vi "电源管理UI.vi"() -> ()   [LabVIEW 2016, in "PLC.lvlib"]
uses:
  PLC.lvlib
  <vilib>/Utility/miscctls.llb/LVPointTypeDef.ctl
panel:
  in  "总氮电源":bool
  in  "CODCr电源":bool
  in  "总磷电源":bool
  in  "氨氮电源":bool
  in  "CODMn电源":bool
  in  "多参数电源":bool
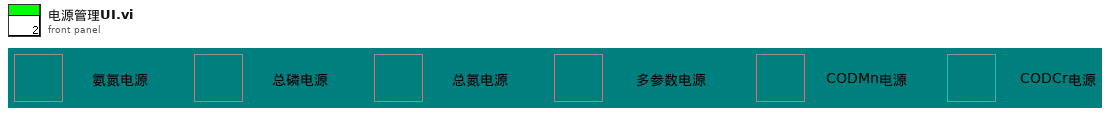
[diagram p1: front panel]
types:
  T1 = typedef "LVPointTypeDef.ctl" = cluster{"Horizontal":i16, "Vertical":i16}
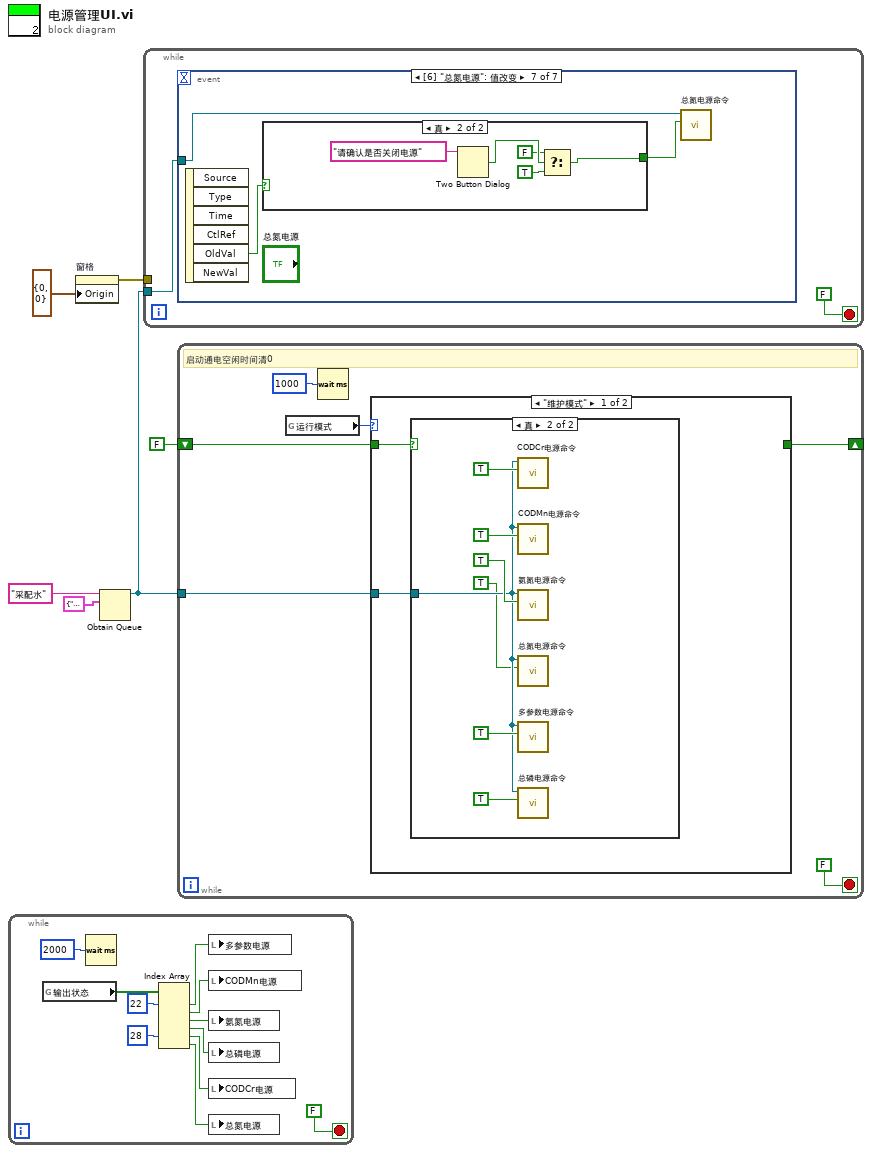
[diagram p0: block diagram]
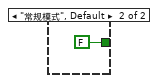
[diagram p3: hidden frame]
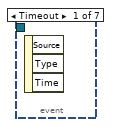
[diagram p4: hidden frame]
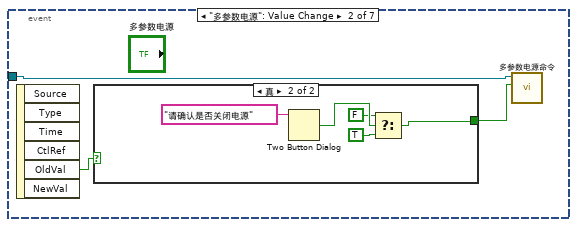
[diagram p5: hidden frame]
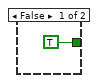
[diagram p6: hidden frame]
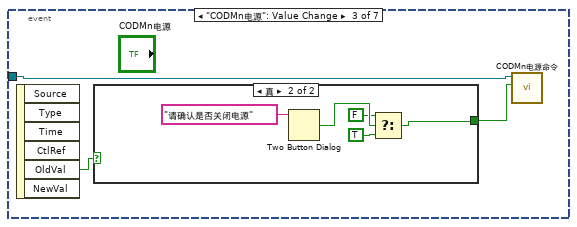
[diagram p7: hidden frame]
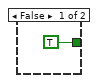
[diagram p8: hidden frame]
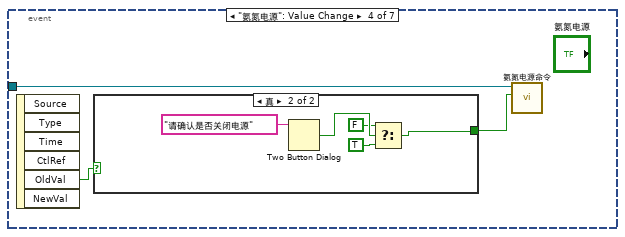
[diagram p9: hidden frame]
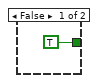
[diagram p10: hidden frame]
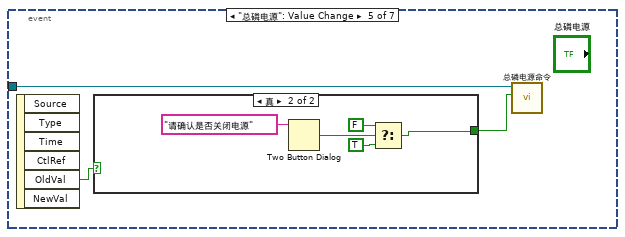
[diagram p11: hidden frame]
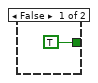
[diagram p12: hidden frame]
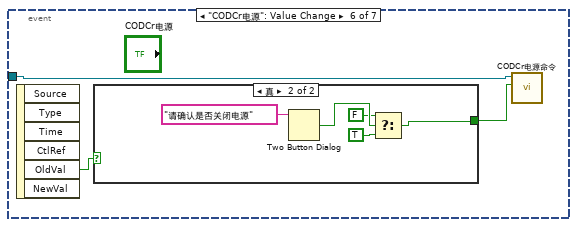
[diagram p13: hidden frame]
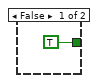
[diagram p14: hidden frame]
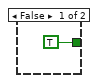
[diagram p15: hidden frame]
diagram:
  n1 = while {
    stop <- FALSE stop-if-true
    n2 = global read "采配水全局变量.vi" "输出状态"() -> (w15:bool[])
    n3 = Wait (ms)(milliseconds to wait=u32 2000 ("等待时间（毫秒）")) -> ()  [unwired: 1 out]
    n4 = Index Array(array=w15, index #1=22 ("索引"), index #5=28 ("索引")) -> (element #1=w10:bool, element #2=w13:bool, element #3=w12:bool, element #4=w11:bool, element #5=w8:bool, element #6=w7:bool)  [unwired: 4 in]
    n5 = local write "多参数电源"(w10) -> ()
    n6 = local write "CODMn电源"(w13) -> ()
    n7 = local write "氨氮电源"(w12) -> ()
    n8 = local write "总磷电源"(w11) -> ()
    n9 = local write "CODCr电源"(w8) -> ()
    n10 = local write "总氮电源"(w7) -> ()
  }
  n11 = property on="窗格" class="Pane"("Origin"=T1 {"Horizontal"=0, "Vertical"=0} ("原点")) -> (error out=w3:errorcluster)  [unwired: 2 in, 1 out]
  n12 = Obtain Queue(name (unnamed)="采配水" ("名称（未命名）"), element data type=cluster{"命令":string, "数据":variant} {"命令"="", "数据"=variant}) -> (queue out=w2:refnum<queue>)  [unwired: 3 in, 2 out]
  n13 = while {
    tunnel: w2 -> [w18]
    tunnel: w3 -> [_]
    stop <- FALSE stop-if-true
    n14 = event shown="[6] \"总氮电源\": 值改变" {
      selector: _ -> [_ _ _ _ _ _ _]
      dyn-events: _ -> [_ _ _ _ _ _ _]
      timeout: _ -> [_ _ _ _ _ _ _]
      tunnel: w18 -> [_ w22 w31 w40 w49 w58 w67]
      event Timeout {
        n15 = event-data() -> ()  [unwired: 1 in, 3 out]
      }
      event "多参数电源": Value Change {
        n16 = event-data() -> ("OldVal"=w21:bool)  [unwired: 1 in, 5 out]
        n17 = case shown="真" w21 {
          tunnel: [TRUE ("T button?") w24] -> w20
          frame False {
          }
          frame True {
            n18 = Two Button Dialog(message="请确认是否关闭电源" ("消息")) -> (T button?=w27:bool)  [unwired: 2 in]
            n19 = Select(t=FALSE, s=w27, f=TRUE ("T button?")) -> (s? t:f=w24:bool)
          }
        }
        n20 = call "多参数电源命令.vi"("通电/断电"=w20, "队列"=w22) -> ()  [unwired: 9 in, 1 out]
      }
      event "CODMn电源": Value Change {
        n21 = event-data() -> ("OldVal"=w30:bool)  [unwired: 1 in, 5 out]
        n22 = case shown="真" w30 {
          tunnel: [TRUE ("T button?") w33] -> w29
          frame False {
          }
          frame True {
            n23 = Two Button Dialog(message="请确认是否关闭电源" ("消息")) -> (T button?=w36:bool)  [unwired: 2 in]
            n24 = Select(t=FALSE, s=w36, f=TRUE ("T button?")) -> (s? t:f=w33:bool)
          }
        }
        n25 = call "CODMn电源命令.vi"("通电/断电"=w29, "队列"=w31) -> ()  [unwired: 9 in, 1 out]
      }
      event "氨氮电源": Value Change {
        n26 = event-data() -> ("OldVal"=w39:bool)  [unwired: 1 in, 5 out]
        n27 = case shown="真" w39 {
          tunnel: [TRUE ("T button?") w42] -> w38
          frame False {
          }
          frame True {
            n28 = Two Button Dialog(message="请确认是否关闭电源" ("消息")) -> (T button?=w45:bool)  [unwired: 2 in]
            n29 = Select(t=FALSE, s=w45, f=TRUE ("T button?")) -> (s? t:f=w42:bool)
          }
        }
        n30 = call "氨氮电源命令.vi"("通电/断电"=w38, "队列"=w40) -> ()  [unwired: 9 in, 1 out]
      }
      event "总磷电源": Value Change {
        n31 = event-data() -> ("OldVal"=w48:bool)  [unwired: 1 in, 5 out]
        n32 = case shown="真" w48 {
          tunnel: [TRUE ("T button?") w51] -> w47
          frame False {
          }
          frame True {
            n33 = Two Button Dialog(message="请确认是否关闭电源" ("消息")) -> (T button?=w54:bool)  [unwired: 2 in]
            n34 = Select(t=FALSE, s=w54, f=TRUE ("T button?")) -> (s? t:f=w51:bool)
          }
        }
        n35 = call "总磷电源命令.vi"("通电/断电"=w47, "队列"=w49) -> ()  [unwired: 9 in, 1 out]
      }
      event "CODCr电源": Value Change {
        n36 = event-data() -> ("OldVal"=w57:bool)  [unwired: 1 in, 5 out]
        n37 = case shown="真" w57 {
          tunnel: [TRUE ("T button?") w60] -> w56
          frame False {
          }
          frame True {
            n38 = Two Button Dialog(message="请确认是否关闭电源" ("消息")) -> (T button?=w63:bool)  [unwired: 2 in]
            n39 = Select(t=FALSE, s=w63, f=TRUE ("T button?")) -> (s? t:f=w60:bool)
          }
        }
        n40 = call "CODCr电源命令.vi"("通电/断电"=w56, "队列"=w58) -> ()  [unwired: 9 in, 1 out]
      }
      event "总氮电源": Value Change {
        n41 = event-data() -> ("OldVal"=w65:bool)  [unwired: 1 in, 5 out]
        n42 = case shown="真" w65 {
          tunnel: [TRUE ("T button?") w69] -> w66
          frame False {
          }
          frame True {
            n43 = Two Button Dialog(message="请确认是否关闭电源" ("消息")) -> (T button?=w72:bool)  [unwired: 2 in]
            n44 = Select(t=FALSE, s=w72, f=TRUE ("T button?")) -> (s? t:f=w69:bool)
          }
        }
        n45 = call "总氮电源命令.vi"("通电/断电"=w66, "队列"=w67) -> ()  [unwired: 9 in, 1 out]
      }
    }
  }
  n46 = while {
    tunnel: w2 -> [w77]
    shift-right: [w74] -> _
    shift-left: FALSE -> [w75]
    stop <- FALSE stop-if-true
    # "启动通电空闲时间清0"
    n47 = global read "系统设置全局变量.vi" "运行模式"() -> (w76:enum16{"维护模式", "常规模式", "应急模式", "质控模式"})
    n48 = Wait (ms)(milliseconds to wait=u32 1000 ("等待时间（毫秒）")) -> ()  [unwired: 1 out]
    n49 = case shown="\"维护模式\"" w76 {
      tunnel: w77 -> [w81 _]
      tunnel: w75 -> [w80 _]
      tunnel: [_ FALSE] -> w74
      frame "维护模式" {
        n50 = case shown="真" w80 {
          tunnel: w81 -> [_ w83]
          frame False {
          }
          frame True {
            n51 = call "CODCr电源命令.vi"("通电/断电"=TRUE, "队列"=w83) -> ()  [unwired: 9 in, 1 out]
            n52 = call "CODMn电源命令.vi"("通电/断电"=TRUE, "队列"=w83) -> ()  [unwired: 9 in, 1 out]
            n53 = call "氨氮电源命令.vi"("通电/断电"=TRUE, "队列"=w83) -> ()  [unwired: 9 in, 1 out]
            n54 = call "总氮电源命令.vi"("通电/断电"=TRUE, "队列"=w83) -> ()  [unwired: 9 in, 1 out]
            n55 = call "多参数电源命令.vi"("通电/断电"=TRUE, "队列"=w83) -> ()  [unwired: 9 in, 1 out]
            n56 = call "总磷电源命令.vi"("通电/断电"=TRUE, "队列"=w83) -> ()  [unwired: 9 in, 1 out]
          }
        }
      }
      frame "常规模式", Default {
      }
    }
  }
